vi "AMZ_S3_APIHLP_Convert Bucket ACL Permission String to Enum.vi"(4 "Permission String":string) -> (1 "Permission":T1)   [LabVIEW 2015, in "LV Interface for Amazon S3.lvlib"]
doc: "Convert the Permission represented as a String to the Enum typedef representation."
uses:
  LV Interface for Amazon S3.lvlib
  Typedefs/AMZ_S3_API_Bucket ACL Permission.ctl
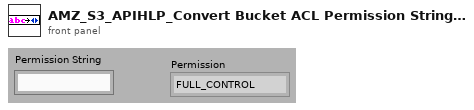
[diagram p1: front panel]
types:
  T1 = typedef "LV Interface for Amazon S3.lvlib/AMZ_S3_API_Bucket ACL Permission.ctl" = enum16{"FULL_CONTROL", "WRITE", "WRITE_ACP", "READ", "READ_ACP"}
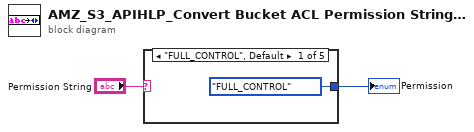
[diagram p0: block diagram]
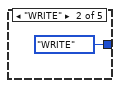
[diagram p2: hidden frame]
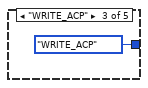
[diagram p3: hidden frame]
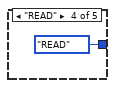
[diagram p4: hidden frame]
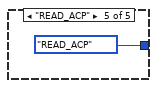
[diagram p5: hidden frame]
diagram:
  n1 = case shown="\"FULL_CONTROL\", Default" "Permission String" {
    tunnel: [AMZ_S3_API_Bucket_ACL_Permission."FULL_CONTROL" ("Permission") AMZ_S3_API_Bucket_ACL_Permission."WRITE" ("Permission") AMZ_S3_API_Bucket_ACL_Permission."WRITE_ACP" ("Permission") AMZ_S3_API_Bucket_ACL_Permission."READ" ("Permission") AMZ_S3_API_Bucket_ACL_Permission."READ_ACP" ("Permission")] -> w1
    frame "FULL_CONTROL", Default {
    }
    frame "WRITE" {
    }
    frame "WRITE_ACP" {
    }
    frame "READ" {
    }
    frame "READ_ACP" {
    }
  }
  "Permission" <- w1
